vi "SMTP Email MIME Send Data Attachment.vi"(4 "MIME content-type":string, 5 "translit":string, 6 "binary (F)":bool, 7 "character set":string, 8 "error in (no error)":errorcluster, 9 "name":string, 10 "data":string, 11 "smtp session":T1) -> (0 "error out":errorcluster, 3 "smtp session out":T1)   [LabVIEW 2009, in "NewNI_SMTPEmail.lvlib"]
uses:
  NewNI_SMTPEmail.lvlib
  SMTP Email Session.ctl
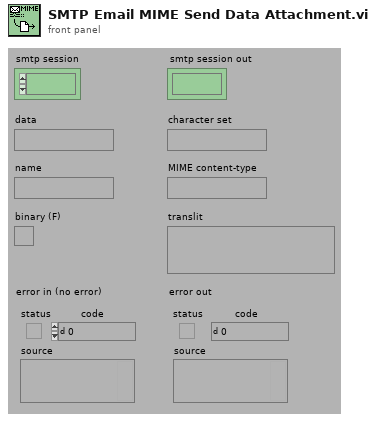
[diagram p1: front panel]
types:
  T1 = typedef "NewNI_SMTPEmail.lvlib/SMTP Email Session.ctl" = refnum<k1>
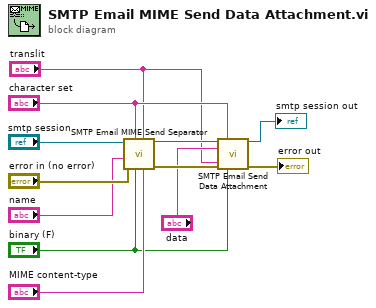
[diagram p0: block diagram]
diagram:
  n1 = call "SMTP Email MIME Send Separator.vi"("MIME content-type"="MIME content-type", "translit"="translit", "binary (F)"="binary (F)", "character set"="character set", "error in (no error)"="error in (no error)", "name"="name", "smtp session"="smtp session") -> ("error out"=w8:errorcluster, "smtp session out"=w7:T1)  [unwired: 1 in, 2 out]
  n2 = call "SMTP Email Send Data Attachment.vi"("smtp session"=w7, "character set"="character set", "data"="data", "error in (no error)"=w8, "binary (F)"="binary (F)", "translit"="translit") -> ("smtp session out"=→"smtp session out":T1, "error out"=→"error out":errorcluster)  [unwired: 8 out]
